vi "Derivative Fletcher.vi"(2 "xi":dbl[](array[numeric]) format="%.2f", 3 "p":dbl[](array[numeric]) format="%.2f", 6 "Parsed Formula":cluster{"table":i32[][], "result":dbl[]}, 7 "Variables":i32[](array[numeric])=[0, 0], 8 "ftol":dbl=0.0001 format="%.2e", 9 "c (start)":dbl=1.0 format="%.2f", 10 "b (start)":dbl=0.5 format="%.2f", 11 "a (start)":dbl format="%.2f") -> (0 "minimum":dbl format="%.2f", 1 "x":dbl format="%.2f")   [LabVIEW 2017, in "NI_Gmath.lvlib"]
uses:
  <vilib>/gmath/NI_Gmath.lvlib
  <vilib>/Analysis/baseanly.llb/Unit Vector (DBL).vi
  <vilib>/Analysis/baseanly.llb/Real Dot Product.vi
  <vilib>/Analysis/NI_AALBase.lvlib
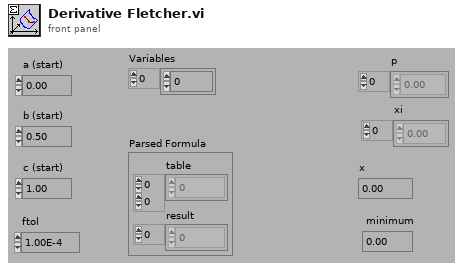
[diagram p1: front panel]
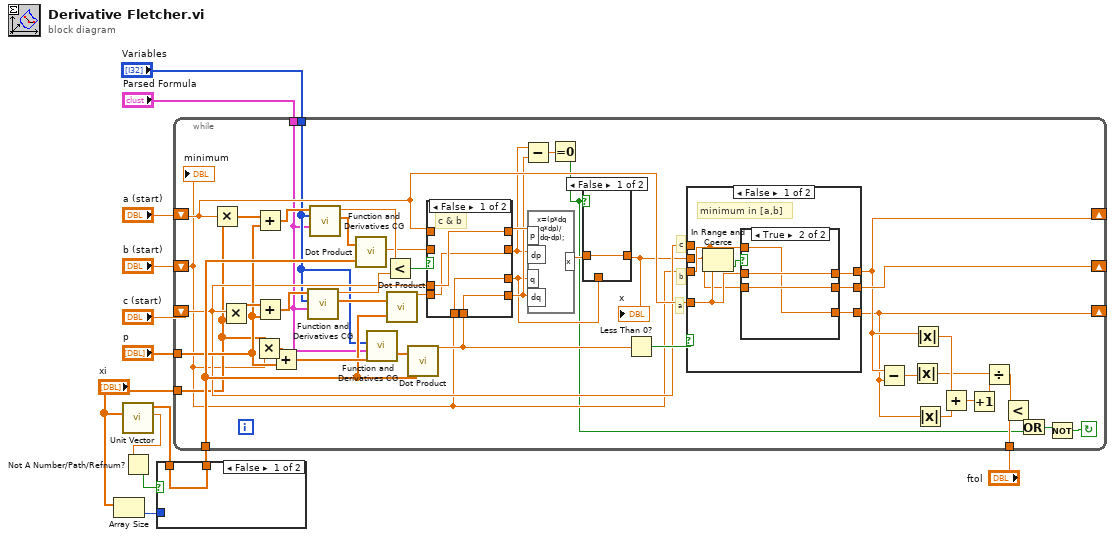
[diagram p0: block diagram]
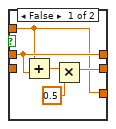
[diagram p4: hidden frame]
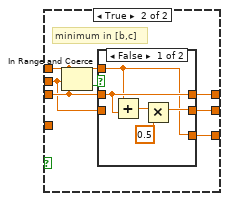
[diagram p5: hidden frame]
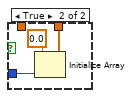
[diagram p7: hidden frame]
diagram:
  n1 = Array Size(array="xi") -> (size(s)=w4:i32)
  n2 = call-poly <vilib>:"Unit Vector.vi"("Input Vector"="xi") -> ("norm"=w7:dbl, "Unit Vector"=w6:dbl[])  [unwired: 8 in, 1 out]
  n3 = Not A Number/Path/Refnum?(number/path/refnum=w7) -> (NaN/Path/Refnum?=w8:bool)
  n4 = case shown="False" w8 {
    tunnel: w6 -> [w14 _]
    tunnel: [w14 w15] -> w3
    tunnel: w4 -> [_ w16]
    frame False {
    }
    frame True {
      n5 = Initialize Array(0.0, w16) -> (w15:dbl[])
    }
  }
  n6 = while {
    tunnel: w3 -> [w37]
    tunnel: "p" -> [w35]
    tunnel: "xi" -> [w33]
    tunnel: "ftol" -> [w50]
    shift-left: "c (start)" -> [w34]
    shift-right: [w57] -> _
    shift-left: "b (start)" -> [w31]
    shift-right: [w59] -> _
    shift-left: "a (start)" -> [w48]
    shift-right: [w58] -> _
    tunnel: "Parsed Formula" -> [w18]
    tunnel: "Variables" -> [w19]
    stop <- w21 continue-if-true
    # "a"
    # "b"
    # "c"
    n7 = Multiply(x=w48, y=w33) -> (x*y=w47:dbl[])
    n8 = Multiply(x=w34, y=w33) -> (x*y=w36:dbl[])
    n9 = Multiply(x=w33, y=w31) -> (x*y=w43:dbl[])
    n10 = Add(x=w47, y=w35) -> (x+y=w46:dbl[])
    n11 = Add(x=w36, y=w35) -> (x+y=w32:dbl[])
    n12 = Add(x=w43, y=w35) -> (x+y=w41:dbl[])
    n13 = call <vilib>:"Function and Derivatives CG.vi"("Parsed Formula"=w18, "Variables"=w19, "X"=w32) -> ("df/dX"=w38:dbl[], "f(X)"=w62:dbl)  [unwired: 7 in]
    n14 = call <vilib>:"Function and Derivatives CG.vi"("Parsed Formula"=w18, "Variables"=w19, "X"=w46) -> ("df/dX"=w45:dbl[], "f(X)"=w63:dbl)  [unwired: 7 in]
    n15 = call-poly <vilib>:"Dot Product.vi"("Y Vector"=w37, "X Vector"=w45) -> ("X * Y"=w44:dbl)  [unwired: 1 out]
    n16 = call <vilib>:"Function and Derivatives CG.vi"("Parsed Formula"=w18, "Variables"=w19, "X"=w41) -> ("df/dX"=w42:dbl[])  [unwired: 7 in, 1 out]
    n17 = Less?(x=w63, y=w62) -> (x < y?=w61:bool)
    n18 = call-poly <vilib>:"Dot Product.vi"("Y Vector"=w37, "X Vector"=w38) -> ("X * Y"=w39:dbl)  [unwired: 1 out]
    n19 = call-poly <vilib>:"Dot Product.vi"("Y Vector"=w37, "X Vector"=w42) -> ("X * Y"=w40:dbl)  [unwired: 1 out]
    n20 = case shown="False" w61 {
      tunnel: w34 -> [w67 _]
      tunnel: w40 -> [w68 w70]
      tunnel: w39 -> [w66 _]
      tunnel: w44 -> [_ w72]
      tunnel: w48 -> [_ w73]
      tunnel: [w67 w73] -> w30
      tunnel: [w66 w72] -> w28
      tunnel: w31 -> [w69 w71]
      tunnel: [w69 w71] -> w24
      tunnel: [w68 w70] -> w29
      frame False {
        # "c & b"
      }
      frame True {
        # "a & b"
      }
    }
    n21 = Subtract(x=w28, y=w29) -> (x-y=w27:dbl)
    n22 = formula code="x=(p*dq-q*dp)/(dq-dp);"("p"=w30, "q"=w24, "dp"=w28, "dq"=w29) -> ("x"=w26:dbl)
    n23 = Equal To 0?(x=w27) -> (x = 0?=w22:bool)
    n24 = case shown="False" w22 {
      tunnel: w26 -> [w64 _]
      tunnel: [w64 w65] -> w25
      tunnel: w24 -> [_ w65]
      frame False {
      }
      frame True {
      }
    }
    "x" <- w25
    n25 = Less Than 0?(x=w40) -> (x < 0?=w60:bool)
    n26 = case shown="False" w60 {
      tunnel: w25 -> [w76 w92]
      tunnel: w31 -> [w79 w94]
      tunnel: w34 -> [_ w90]
      tunnel: w48 -> [w77 _]
      tunnel: [w78 w93] -> w58
      tunnel: [w75 w91] -> w59
      tunnel: [w74 w89] -> w57
      frame False {
        # "minimum in [a,b]"
        n27 = In Range and Coerce(upper limit=w79, x=w76, lower limit=w77) -> (In Range?=w80:bool)  [unwired: 1 out]
        n28 = case shown="True" w80 {
          tunnel: w77 -> [w83 w88]
          tunnel: [w83 w88] -> w78
          tunnel: w76 -> [_ w87]
          tunnel: [w82 w87] -> w75
          tunnel: w79 -> [w81 w86]
          tunnel: [w81 w86] -> w74
          frame False {
            n29 = Add(x=w81, y=w83) -> (x+y=w85:dbl)
            n30 = Multiply(x=w85, y=0.5) -> (x*y=w82:dbl)
          }
          frame True {
          }
        }
      }
      frame True {
        # "minimum in [b,c]"
        n31 = In Range and Coerce(upper limit=w90, x=w92, lower limit=w94) -> (In Range?=w95:bool)  [unwired: 1 out]
        n32 = case shown="False" w95 {
          tunnel: w94 -> [w98 w103]
          tunnel: [w98 w103] -> w93
          tunnel: w92 -> [_ w102]
          tunnel: [w97 w102] -> w91
          tunnel: w90 -> [w96 w101]
          tunnel: [w96 w101] -> w89
          frame False {
            n33 = Add(x=w96, y=w98) -> (x+y=w100:dbl)
            n34 = Multiply(x=w100, y=0.5) -> (x*y=w97:dbl)
          }
          frame True {
          }
        }
      }
    }
    n35 = Subtract(x=w58, y=w57) -> (x-y=w49:dbl)
    n36 = Absolute Value(x=w49) -> (abs(x)=w52:dbl)
    n37 = Absolute Value(x=w58) -> (abs(x)=w56:dbl)
    n38 = Absolute Value(x=w57) -> (abs(x)=w55:dbl)
    n39 = Add(x=w56, y=w55) -> (x+y=w54:dbl)
    n40 = Increment(x=w54) -> (x+1=w53:dbl)
    n41 = Divide(x=w52, y=w53) -> (x/y=w51:dbl)
    n42 = Less?(x=w51, y=w50) -> (x < y?=w23:bool)
    n43 = Or(x=w23, y=w22) -> (x .or. y?=w20:bool)
    n44 = Not(x=w20) -> (.not. x?=w21:bool)
    "minimum" <- w31
  }
